vi "Create.vi"   [LabVIEW 2018, in "Toolkit.lvlib" / "KnownHost.lvclass"]
uses:
  KnownHost.lvclass
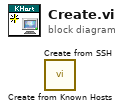
[diagram p0: block diagram]
diagram:
  n1 = call "Create from Known Hosts.vi"() -> ()  [unwired: 10 in, 2 out]
  n2 = call "Create from SSH.vi"() -> ()  [unwired: 10 in, 2 out]
